vi "XP2100_Module_Manual Test_Main.vi"() -> ()   [LabVIEW 2013]
doc: "This template is for the Queued Message Handler design pattern.\n\nThe Event Handling Loop generates messages based on user interface actions.\n\nThe Message Handling Loop processes messages generated by the Event Handling Loop, or by other messages. The messages are string values, so new messages can be added easily to the Message Cases case structure in the Message Handling Loop. Each message cluster can also provide an optional value for Message Data, which is a variant that can be converted to whatever message-specific data is required."
uses:
  <instrlib>/niHSDIO/niHSDIO.llb/niHSDIO_ctl Voltage Logic Family Values (Ring).ctl
  <instrlib>/niDCPower/nidcpower.llb/niDCPower Sense.ctl
  Controls/Reg_Address_Data.ctl
  Controls/USID.ctl
  controls/UI Data.ctl
  support/Message Queue/Enqueue Message (Single).vi
  support/Message Queue/Enqueue Message (Array).vi
  <vilib>/Utility/error.llb/Error Cluster From Error Code.vi
  <vilib>/ErrorRing/Error Ring.xnode
  support/Message Queue/Message Queue.lvlib
  support/User Event - Stop/User Event - Stop.lvlib
panel:
  in  "Measure":bool=TRUE
  in  "Tab Control":T1(tab)
  in  "DUT and Bridge SMU Settings":T3={"SMU Settings"={"CH"={"voltage level range"=6.0, "current limit"=0.1, "current limit range"=0.1, "voltage level "=1.8, "CH_VIO_BRIDGE"="0", "Output Enabled"=TRUE}, "CH 2"={"voltage level range"=6.0, "current limit"=0.1, "current limit range"=0.1, "voltage level "=1.8, "CH_VSU"="1", "Output Enabled"=TRUE}, "CH 3"={"voltage level range"=6.0, "current limit"=0.1, "current limit range"=0.1, "voltage level "=1.8, "CH_RFC"="2", "Output Enabled"=TRUE}, "CH 4"={"voltage level range"=6.0, "current limit"=0.1, "current limit range"=0.1, "voltage level "=1.8, "CH_NA"="3", "Output Enabled"=FALSE}}, "sense"=1008, "aperture time"=0.01666} {"aperture time" format="%.2p"; "sense" items=["Local"=1008, "Remote"=1009]; "SMU Settings"."CH 4"."voltage level" format="%#.6p"; "SMU Settings"."CH 4"."current limit range" format="%#.6p"; "SMU Settings"."CH 4"."current limit" format="%#.6p"; "SMU Settings"."CH 4"."voltage level range" format="%#.6p"; "SMU Settings"."CH 3"."voltage level" format="%#.6p"; "SMU Settings"."CH 3"."current limit range" format="%#.6p"; "SMU Settings"."CH 3"."current limit" format="%#.6p"; "SMU Settings"."CH 3"."voltage level range" format="%#.6p"; "SMU Settings"."CH 2"."voltage level" format="%#.6p"; "SMU Settings"."CH 2"."current limit range" format="%#.6p"; "SMU Settings"."CH 2"."current limit" format="%#.6p"; "SMU Settings"."CH 2"."voltage level range" format="%#.6p"; "SMU Settings"."CH"."voltage level" format="%#.6p"; "SMU Settings"."CH"."current limit range" format="%#.6p"; "SMU Settings"."CH"."current limit" format="%#.6p"; "SMU Settings"."CH"."voltage level range" format="%#.6p"}
  in  "Instrument_Visas":T4={"DUT and Bridge Power"="4145_1", "HV_SMU"="4145_0"}
  in  "HDSIO_Settings":T6={"HSDIO VISA"="6556_0", "Waveform Directory"=path "C:/Users/user/Documents/XP2100/Waveforms", "logic family "=8, "Clock Rate"=20000000.0, "channel list (Clock,Data)"="4,6"} {"Clock Rate" format="%.2p"; "logic family" items=["5.0V Logic"=5, "3.3V Logic"=6, "2.5V Logic"=7, "1.8V Logic"=8, "1.5V Logic"=80, "1.2V Logic"=81]}
  in  "Initialize Instruments":bool
  in  "Update SMU's":bool
  in  "Throw Settings: Source Current":T7={"SMU Settings"={"CH"={"Voltage Limit"=1.0, "current limit"=0.01, "Voltage limit range"=6.0, "Current level"=0.01, "CH_RF1"="0", "Output Enabled"=TRUE}, "CH"={"Voltage Limit"=1.0, "current limit"=0.01, "Voltage limit range"=6.0, "Current level"=0.01, "CH_RF2"="1", "Output Enabled"=TRUE}, "CH"={"Voltage Limit"=1.0, "current limit"=0.01, "Voltage limit range"=6.0, "Current level"=0.01, "CH_RF3"="2", "Output Enabled"=TRUE}, "CH"={"Voltage Limit"=1.0, "current limit"=0.01, "Voltage limit range"=6.0, "Current level"=0.01, "CH_RF4"="3", "Output Enabled"=TRUE}}, "sense"=1009, "aperture time"=0.01666} {"aperture time" format="%.2p"; "sense" items=["Local"=1008, "Remote"=1009]; "SMU Settings"."CH"."Current level" format="%#.6p"; "SMU Settings"."CH"."Voltage limit range" format="%#.6p"; "SMU Settings"."CH"."current limit" format="%#.6p"; "SMU Settings"."CH"."Voltage Limit" format="%#.6p"; "SMU Settings"."CH"."Current level" format="%#.6p"; "SMU Settings"."CH"."Voltage limit range" format="%#.6p"; "SMU Settings"."CH"."current limit" format="%#.6p"; "SMU Settings"."CH"."Voltage Limit" format="%#.6p"; "SMU Settings"."CH"."Current level" format="%#.6p"; "SMU Settings"."CH"."Voltage limit range" format="%#.6p"; "SMU Settings"."CH"."current limit" format="%#.6p"; "SMU Settings"."CH"."Voltage Limit" format="%#.6p"; "SMU Settings"."CH"."Current level" format="%#.6p"; "SMU Settings"."CH"."Voltage limit range" format="%#.6p"; "SMU Settings"."CH"."current limit" format="%#.6p"; "SMU Settings"."CH"."Voltage Limit" format="%#.6p"}
  in  "Test Script w_Triggers":bool
  in  "Test Script":string="Script Lowpower\nWait until scriptTrigger0\nGenerate U13LowPower\nend Script"
  in  "RFFE Function":enum16{"Write", "Read"}(ring)
  in  "Reg_Address_Data":T8={"Address"=81, "Data"=0} {"Data" min=1; "Address" format="%.0x"}
  in  "USID":T9 max=15
  out "Read Data":cluster{"USID":u8, "Register":u8, "Data":u8} {"Register" max=31 format="%.0x"; "USID" max=15}
  in  "Run RFFE Waveform":bool
  out "Ext_Read_Reg":i32[](array[numeric])
  out "Ext_Read_Data":u8[](array[numeric])=[31, 144, 7]
  in  "Run Script":bool
  in  "Script Steps":string="\tGenerate\tBRGu8r1Cd56\n\tWait 20\t\n\tGenerate\tBRGu8r0d13\n\tWait 20\t\n\tGenerate\tBRGu8r4d7\n\tWait 20\t\n\tGenerate\tBRGu8rCd1\n\tWait 20\t\n\tGenerate\tBRGu8r3d46\n\tWait 20\t\n\tGenerate\tBRGu8r2Bd4\n\tWait 20\t\n\tGenerate\tBRGu8r4d103\n\tWait 20\t\n\tGenerate\tBRGu8r2d27\n\tWait 20\t\n\tGenerate\tBRGu8r5d9\n\tWait 20\t\n\tGenerate\tBRGu8r6d187\n\tWait 20\t\n\tGenerate\tBRGu8r7d4\n\tWait 20\t\n\tGenerate\tBRGu8r3d110\n\tWait 20\t\n\tGenerate\tBRGu8r1d184\n\tWait 20\t\n\tGenerate\tBRGu8r80d2\n\tWait 20\t\n\tGenerate\tBRGu8r4Ad242\n\tWait 20\t\n\tGenerate\tBRGu8r4Bd249\n\tWait 20\t\n\tGenerate\tBRGu8r4Dd244\n\tWait 20\t\n\tGenerate\tBRGu8rC1d253\n\twait 20\n\tGenerate \tBRGu2rAd133\n\twait 20\n\tGenerate \tBRGu8r4Dd254\n\twait 20\n\tGenerate \tBRGu8rC1d241\n\twait 20\n\tGenerate \tBRGu8rC1d247\n\twait 400"
  out "Dut and Bridge Measurements":T10 {"current measurements" format="%#_6p"}
  in  "Script Notepad: Initialize Bridge":string="\tGenerate\tBRGu8r1Cd56\n\tWait 20\t\n\tGenerate\tBRGu8r0d13\n\tWait 20\t\n\tGenerate\tBRGu8r4d7\n\tWait 20\t\n\tGenerate\tBRGu8rCd1\n\tWait 20\t\n\tGenerate\tBRGu8r3d46\n\tWait 20\t\n\tGenerate\tBRGu8r2Bd4\n\tWait 20\t\n\tGenerate\tBRGu8r4d103\n\tWait 20\t\n\tGenerate\tBRGu8r2d27\n\tWait 20\t\n\tGenerate\tBRGu8r5d9\n\tWait 20\t\n\tGenerate\tBRGu8r6d187\n\tWait 20\t\n\tGenerate\tBRGu8r7d4\n\tWait 20\t\n\tGenerate\tBRGu8r3d110\n\tWait 20\t\n\tGenerate\tBRGu8r1d184\n\tWait 20\t\n\tGenerate\tBRGu8r80d2\n\tWait 20\t\n\tGenerate\tBRGu8r4Ad242\n\tWait 20\t\n\tGenerate\tBRGu8r4Bd249\n\tWait 20\t\n\tGenerate\tBRGu8r4Dd244\n\tWait 20\t\n\tGenerate\tBRGu8rC1d253\n\twait 20\n\tGenerate \tBRGu2rAd133\n\twait 20\n\tGenerate \tBRGu8r4Dd254\n\twait 20\n\tGenerate \tBRGu8rC1d241\n\twait 20\n\tGenerate \tBRGu8rC1d247\n\twait 400"
  in  "DUT Info":T11={"Lot #"="", "Wafer #"="", "DUT Coordinates"="", "Comments"="generate HV29"}
  in  "Path":path=path "C:/Users/er080167/Desktop/Delete"
  in  "Save Button":bool
  out "USIDs_Detected":u8[](array[numeric])
  in  "Scan USID's":bool
  out "Throw Measurements":T10 {"current measurements" format="%#_6p"}
  out "Throw_Resitances":dbl[](array[numeric]) format="%#_6p"
  out "4_CH_SMU_Settings_Readback":T12(array[cluster]) {"sense 2" items=["Local"=1008, "Remote"=1009]}
  out "Write or Read":digitalwaveform(graph)={"t0"=timestamp(3585852840.1106524 s since 1904-01-01), "dt"=5e-07, "Y"={"transitions"=[], "data"=[[1, 0, 1, 0], [1, 0, 1, 0], [1, 0, 1, 0], [1, 0, 1, 0], [1, 0, 1, 0], [1, 0, 1, 0], [1, 0, 1, 0], [1, 0, 1, 0], [0, 0, 0, 0], [0, 0, 0, 0], [0, 0, 0, 0], [0, 0, 0, 0], [0, 0, 0, 0], [0, 0, 0, 0], [0, 0, 0, 0], [0, 0, 0, 0], [0, 1, 0, 1], [0, 1, 0, 1], [0, 1, 0, 1], [0, 1, 0, 1], [0, 0, 0, 0], [0, 0, 0, 0], [0, 0, 0, 0], [0, 0, 0, 0], [1, 1, 1, 1], [1, 1, 1, 1], [1, 1, 1, 1], [1, 1, 1, 1], [1, 0, 1, 0], [1, 0, 1, 0], [1, 0, 1, 0], [1, 0, 1, 0], [1, 1, 1, 1], [1, 1, 1, 1], [1, 1, 1, 1], [1, 1, 1, 1], [1, 0, 1, 0], [1, 0, 1, 0], [1, 0, 1, 0], [1, 0, 1, 0], [0, 1, 0, 1], [0, 1, 0, 1], [0, 1, 0, 1], [0, 1, 0, 1], [0, 0, 0, 0], [0, 0, 0, 0], [0, 0, 0, 0], [0, 0, 0, 0], [0, 1, 0, 1], [0, 1, 0, 1], [0, 1, 0, 1], [0, 1, 0, 1], [0, 0, 0, 0], [0, 0, 0, 0], [0, 0, 0, 0], [0, 0, 0, 0], [1, 1, 1, 1], [1, 1, 1, 1], [1, 1, 1, 1], [1, 1, 1, 1], [1, 0, 1, 0], [1, 0, 1, 0], [1, 0, 1, 0], [1, 0, 1, 0], [0, 1, 0, 1], [0, 1, 0, 1], [0, 1, 0, 1], [0, 1, 0, 1], [0, 0, 0, 0], [0, 0, 0, 0], [0, 0, 0, 0], [0, 0, 0, 0], [1, 1, 1, 1], [1, 1, 1, 1], [1, 1, 1, 1], [1, 1, 1, 1], [1, 0, 1, 0], [1, 0, 1, 0], [1, 0, 1, 0], [1, 0, 1, 0], [1, 1, 1, 1], [1, 1, 1, 1], [1, 1, 1, 1], [1, 1, 1, 1], [1, 0, 1, 0], [1, 0, 1, 0], [1, 0, 1, 0], [1, 0, 1, 0], [1, 1, 1, 1], [1, 1, 1, 1], [1, 1, 1, 1], [1, 1, 1, 1], [1, 0, 1, 0], [1, 0, 1, 0], [1, 0, 1, 0], [1, 0, 1, 0], [0, 1, 0, 1], [0, 1, 0, 1], [0, 1, 0, 1], [0, 1, 0, 1], [0, 0, 0, 0], [0, 0, 0, 0], [0, 0, 0, 0], [0, 0, 0, 0], [0, 1, 0, 1], [0, 1, 0, 1], [0, 1, 0, 1], [0, 1, 0, 1], [0, 0, 0, 0], [0, 0, 0, 0], [0, 0, 0, 0], [0, 0, 0, 0], [1, 1, 1, 1], [1, 1, 1, 1], [1, 1, 1, 1], [1, 1, 1, 1], [1, 0, 1, 0], [1, 0, 1, 0], [1, 0, 1, 0], [1, 0, 1, 0], [1, 1, 1, 1], [1, 1, 1, 1], [1, 1, 1, 1], [1, 1, 1, 1], [1, 0, 1, 0], [1, 0, 1, 0], [1, 0, 1, 0], [1, 0, 1, 0], [0, 1, 0, 1], [0, 1, 0, 1], [0, 1, 0, 1], [0, 1, 0, 1], [0, 0, 0, 0], [0, 0, 0, 0], [0, 0, 0, 0], [0, 0, 0, 0], [0, 1, 0, 1], [0, 1, 0, 1], [0, 1, 0, 1], [0, 1, 0, 1], [0, 0, 0, 0], [0, 0, 0, 0], [0, 0, 0, 0], [0, 0, 0, 0], [0, 1, 0, 1], [0, 1, 0, 1], [0, 1, 0, 1], [0, 1, 0, 1], [0, 0, 0, 0], [0, 0, 0, 0], [0, 0, 0, 0], [0, 0, 0, 0], [0, 1, 0, 1], [0, 1, 0, 1], [0, 1, 0, 1], [0, 1, 0, 1], [0, 0, 0, 0], [0, 0, 0, 0], [0, 0, 0, 0], [0, 0, 0, 0], [0, 1, 0, 1], [0, 1, 0, 1], [0, 1, 0, 1], [0, 1, 0, 1], [0, 0, 0, 0], [0, 0, 0, 0], [0, 0, 0, 0], [0, 0, 0, 0], [0, 1, 0, 1], [0, 1, 0, 1], [0, 1, 0, 1], [0, 1, 0, 1], [0, 0, 0, 0], [0, 0, 0, 0], [0, 0, 0, 0], [0, 0, 0, 0], [0, 1, 0, 1], [0, 1, 0, 1], [0, 1, 0, 1], [0, 1, 0, 1], [0, 0, 0, 0], [0, 0, 0, 0], [0, 0, 0, 0], [0, 0, 0, 0], [0, 1, 0, 1], [0, 1, 0, 1], [0, 1, 0, 1], [0, 1, 0, 1], [0, 0, 0, 0], [0, 0, 0, 0], [0, 0, 0, 0], [0, 0, 0, 0], [0, 1, 0, 1], [0, 1, 0, 1], [0, 1, 0, 1], [0, 1, 0, 1], [0, 0, 0, 0], [0, 0, 0, 0], [0, 0, 0, 0], [0, 0, 0, 0], [1, 0, 1, 0], [1, 0, 1, 0], [1, 0, 1, 0], [1, 0, 1, 0], [1, 0, 1, 0], [1, 0, 1, 0], [1, 0, 1, 0], [1, 0, 1, 0], [0, 0, 0, 0], [0, 0, 0, 0], [0, 0, 0, 0], [0, 0, 0, 0], [0, 0, 0, 0], [0, 0, 0, 0], [0, 0, 0, 0], [0, 0, 0, 0], [0, 1, 0, 1], [0, 1, 0, 1], [0, 1, 0, 1], [0, 1, 0, 1], [0, 0, 0, 0], [0, 0, 0, 0], [0, 0, 0, 0], [0, 0, 0, 0], [1, 1, 1, 1], [1, 1, 1, 1], [1, 1, 1, 1], [1, 1, 1, 1], [1, 0, 1, 0], [1, 0, 1, 0], [1, 0, 1, 0], [1, 0, 1, 0], [1, 1, 1, 1], [1, 1, 1, 1], [1, 1, 1, 1], [1, 1, 1, 1], [1, 0, 1, 0], [1, 0, 1, 0], [1, 0, 1, 0], [1, 0, 1, 0], [0, 1, 0, 1], [0, 1, 0, 1], [0, 1, 0, 1], [0, 1, 0, 1], [0, 0, 0, 0], [0, 0, 0, 0], [0, 0, 0, 0], [0, 0, 0, 0], [0, 1, 0, 1], [0, 1, 0, 1], [0, 1, 0, 1], [0, 1, 0, 1], [0, 0, 0, 0], [0, 0, 0, 0], [0, 0, 0, 0], [0, 0, 0, 0], [1, 1, 1, 1], [1, 1, 1, 1], [1, 1, 1, 1], [1, 1, 1, 1], [1, 0, 1, 0], [1, 0, 1, 0], [1, 0, 1, 0], [1, 0, 1, 0], [1, 1, 1, 1], [1, 1, 1, 1], [1, 1, 1, 1], [1, 1, 1, 1], [1, 0, 1, 0], [1, 0, 1, 0], [1, 0, 1, 0], [1, 0, 1, 0], [1, 1, 1, 1], [1, 1, 1, 1], [1, 1, 1, 1], [1, 1, 1, 1], [1, 0, 1, 0], [1, 0, 1, 0], [1, 0, 1, 0], [1, 0, 1, 0], [1, 1, 1, 1], [1, 1, 1, 1], [1, 1, 1, 1], [1, 1, 1, 1], [1, 0, 1, 0], [1, 0, 1, 0], [1, 0, 1, 0], [1, 0, 1, 0], [1, 1, 1, 1], [1, 1, 1, 1], [1, 1, 1, 1], [1, 1, 1, 1], [1, 0, 1, 0], [1, 0, 1, 0], [1, 0, 1, 0], [1, 0, 1, 0], [0, 1, 0, 1], [0, 1, 0, 1], [0, 1, 0, 1], [0, 1, 0, 1], [0, 0, 0, 0], [0, 0, 0, 0], [0, 0, 0, 0], [0, 0, 0, 0], [0, 1, 0, 1], [0, 1, 0, 1], [0, 1, 0, 1], [0, 1, 0, 1], [0, 0, 0, 0], [0, 0, 0, 0], [0, 0, 0, 0], [0, 0, 0, 0], [0, 1, 0, 1], [0, 1, 0, 1], [0, 1, 0, 1], [0, 1, 0, 1], [0, 0, 0, 0], [0, 0, 0, 0], [0, 0, 0, 0], [0, 0, 0, 0], [0, 1, 0, 1], [0, 1, 0, 1], [0, 1, 0, 1], [0, 1, 0, 1], [0, 0, 0, 0], [0, 0, 0, 0], [0, 0, 0, 0], [0, 0, 0, 0], [1, 1, 5, 1], [1, 1, 5, 1], [1, 1, 5, 1], [1, 1, 5, 1], [1, 0, 4, 0], [1, 0, 5, 0], [1, 0, 5, 0], [1, 0, 5, 0], [0, 1, 5, 1], [0, 1, 5, 1], [0, 1, 5, 1], [0, 1, 5, 1], [0, 0, 3, 0], [0, 0, 5, 0], [0, 0, 5, 0], [0, 0, 5, 0], [0, 1, 5, 1], [0, 1, 5, 1], [0, 1, 5, 1], [0, 1, 5, 1], [0, 0, 3, 0], [0, 0, 5, 0], [0, 0, 5, 0], [0, 0, 5, 0], [0, 1, 5, 1], [0, 1, 5, 1], [0, 1, 5, 1], [0, 1, 5, 1], [0, 0, 3, 0], [0, 0, 5, 0], [0, 0, 5, 0], [0, 0, 5, 0], [0, 1, 5, 1], [0, 1, 5, 1], [0, 1, 5, 1], [0, 1, 5, 1], [0, 0, 3, 0], [0, 0, 5, 0], [0, 0, 5, 0], [0, 0, 5, 0], [0, 1, 5, 1], [0, 1, 5, 1], [0, 1, 5, 1], [0, 1, 5, 1], [0, 0, 3, 0], [0, 0, 5, 0], [0, 0, 5, 0], [0, 0, 5, 0], [0, 1, 5, 1], [0, 1, 5, 1], [0, 1, 5, 1], [0, 1, 5, 1], [0, 0, 3, 0], [0, 0, 5, 0], [0, 0, 5, 0], [0, 0, 5, 0], [0, 1, 5, 1], [0, 1, 5, 1], [0, 1, 5, 1], [0, 1, 5, 1], [0, 0, 3, 0], [0, 0, 5, 0], [0, 0, 5, 0], [0, 0, 5, 0], [0, 1, 5, 1], [0, 1, 5, 1], [0, 1, 5, 1], [0, 1, 5, 1], [0, 0, 3, 0], [0, 0, 5, 0], [0, 0, 5, 0], [0, 0, 5, 0], [0, 1, 0, 1], [0, 1, 0, 1], [0, 1, 0, 1], [0, 1, 0, 1], [0, 0, 0, 0], [0, 0, 0, 0], [0, 0, 0, 0], [0, 0, 0, 0]]}}
  out "Throw_4_CH_SMU_Settings_Readback":T12(array[cluster]) {"sense 2" items=["Local"=1008, "Remote"=1009]}
  out "Display <Replace Me>":string="\"Exit\" button pressed"
  in  "Exit":bool
  # "CH_VIO_BRIDGE"
  # "CH_VSU"
  # "CH_RFC"
  # "CH_NA"
  # "CH_VIO_BRIDGE"
  # "CH_VSU"
  # "CH_VP"
  # "CH_DUT_VIO"
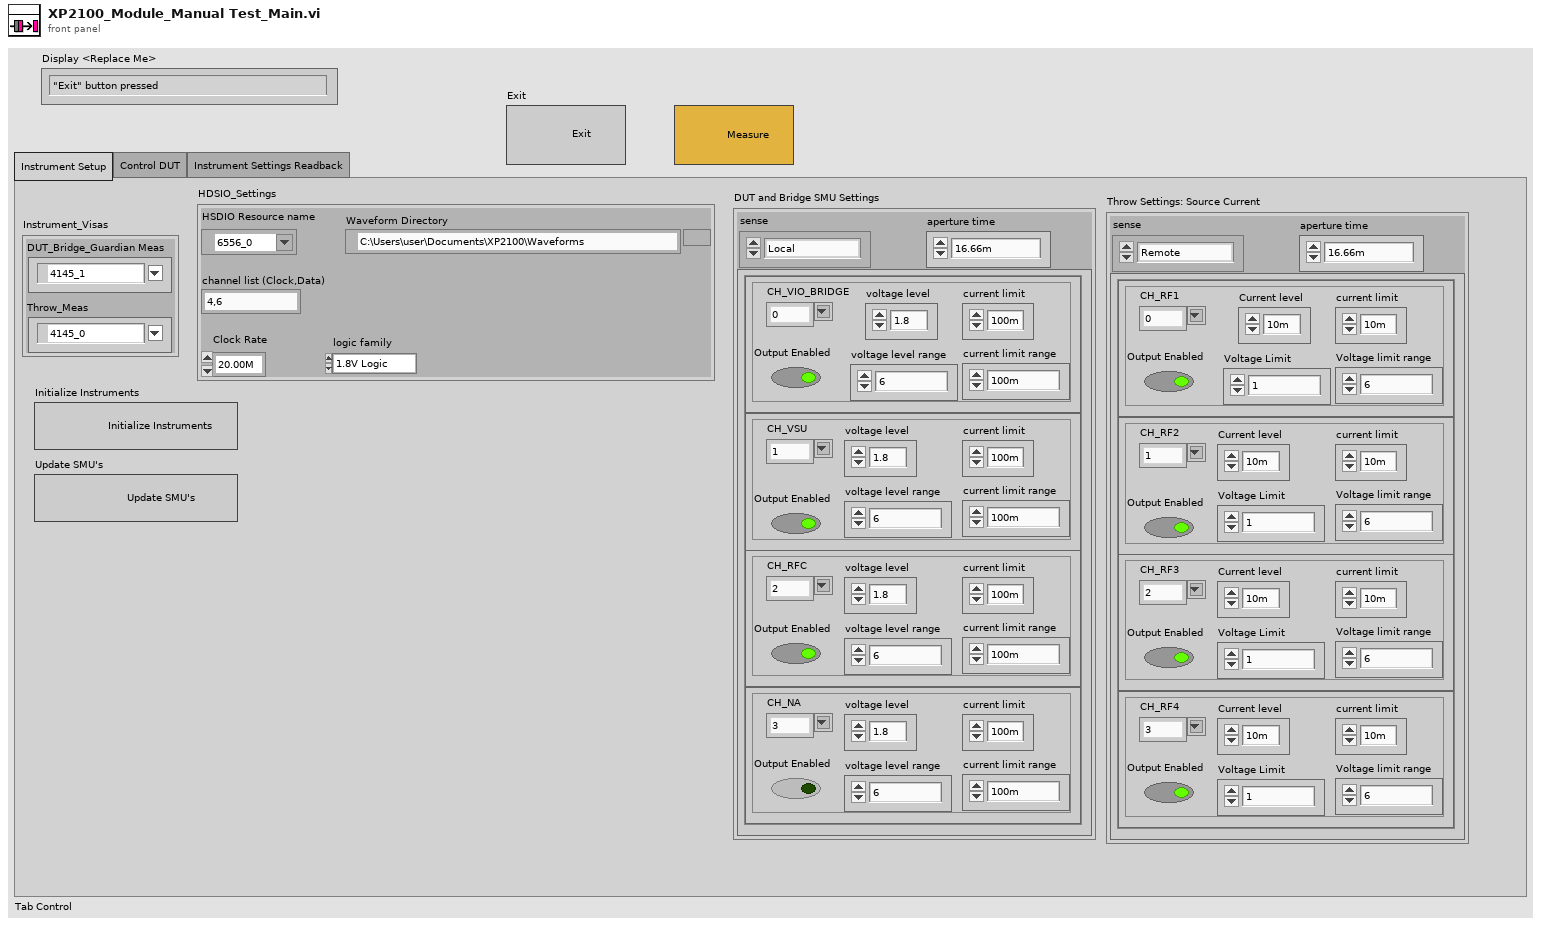
[diagram p1: front panel]
types:
  T1 = enum32{"Instrument Setup", "Control DUT", "Instrument Settings Readback"}
  T2 = typedef "niDCPower Sense.ctl" = i32
  T3 = cluster{"SMU Settings":cluster{"CH":cluster{"voltage level range":dbl, "current limit":dbl, "current limit range":dbl, "voltage level ":dbl, "CH_VIO_BRIDGE":string, "Output Enabled":bool}, "CH 2":cluster{"voltage level range":dbl, "current limit":dbl, "current limit range":dbl, "voltage level ":dbl, "CH_VSU":string, "Output Enabled":bool}, "CH 3":cluster{"voltage level range":dbl, "current limit":dbl, "current limit range":dbl, "voltage level ":dbl, "CH_RFC":string, "Output Enabled":bool}, "CH 4":cluster{"voltage level range":dbl, "current limit":dbl, "current limit range":dbl, "voltage level ":dbl, "CH_NA":string, "Output Enabled":bool}}, "sense":T2, "aperture time":dbl}
  T4 = cluster{"DUT and Bridge Power":refnum<k15>, "HV_SMU":refnum<k15>}
  T5 = typedef "niHSDIO_ctl Voltage Logic Family Values (Ring).ctl" = i32
  T6 = cluster{"HSDIO VISA":refnum<k15>, "Waveform Directory":path, "logic family ":T5, "Clock Rate":dbl, "channel list (Clock,Data)":string}
  T7 = cluster{"SMU Settings":cluster{"CH":cluster{"Voltage Limit":dbl, "current limit":dbl, "Voltage limit range":dbl, "Current level":dbl, "CH_RF1":string, "Output Enabled":bool}, "CH":cluster{"Voltage Limit":dbl, "current limit":dbl, "Voltage limit range":dbl, "Current level":dbl, "CH_RF2":string, "Output Enabled":bool}, "CH":cluster{"Voltage Limit":dbl, "current limit":dbl, "Voltage limit range":dbl, "Current level":dbl, "CH_RF3":string, "Output Enabled":bool}, "CH":cluster{"Voltage Limit":dbl, "current limit":dbl, "Voltage limit range":dbl, "Current level":dbl, "CH_RF4":string, "Output Enabled":bool}}, "sense":T2, "aperture time":dbl}
  T8 = typedef "Reg_Address_Data.ctl" = cluster{"Address":u8, "Data":u8}
  T9 = typedef "USID.ctl" = u8
  T10 = cluster{"voltage measurements":dbl[], "current measurements":dbl[]}
  T11 = cluster{"Lot #":string, "Wafer #":string, "DUT Coordinates":string, "Comments":string}
  T12 = cluster{"Source Range":dbl, "Source Limit":dbl, "Source  limit range":dbl, "Source level":dbl, "CH":string, "Output Enabled":bool, "Source Mode":enum16{"Voltage", "Current"}, "aperture time":dbl, "sense 2":T2}[]
  T13 = cluster{"HV SMU Settings":cluster{"Source Range":dbl, "Source Limit":dbl, "Source  limit range":dbl, "Source level":dbl, "CH":string, "Output Enabled":bool, "Source Mode":enum16{"Voltage", "Current"}, "aperture time":dbl, "sense 2":T2}, "PI<0>":cluster{"Source Range":dbl, "Source Limit":dbl, "Source  limit range":dbl, "Source level":dbl, "CH":string, "Output Enabled":bool, "Source Mode":enum16{"Voltage", "Current"}, "aperture time":dbl, "sense 2":T2}}
  T14 = cluster{"SMU Settings":cluster{"CH":cluster{"voltage level range":dbl, "current limit":dbl, "current limit range":dbl, "voltage level ":dbl, "CH_VIO_BRIDGE":string, "Output Enabled":bool}, "CH 2":cluster{"voltage level range":dbl, "current limit":dbl, "current limit range":dbl, "voltage level ":dbl, "CH_VSU":string, "Output Enabled":bool}, "CH 3":cluster{"voltage level range":dbl, "current limit":dbl, "current limit range":dbl, "voltage level ":dbl, "CH_VP":string, "Output Enabled":bool}, "CH 4":cluster{"voltage level range":dbl, "current limit":dbl, "current limit range":dbl, "voltage level ":dbl, "CH_DUT_VIO":string, "Output Enabled":bool}}, "sense":T2, "aperture time":dbl}
  T15 = cluster{"HSDIO_ACQ":refnum<k15>, "HSDIO_GEN":refnum<k15>}
  T16 = typedef "UI Data.ctl" = cluster{"Boolean <Replace Me>":bool, "String <Replace Me>":string, "Numeric <Replace Me>":dbl, "Do Something Ref":refnum<vi>, "Do Something Else Ref":refnum<vi>, "Data Display Ref":refnum<vi>, "Exit Button Ref":refnum<vi>}
  T17 = typedef "Message Queue.lvlib/All Message Queues.ctl" = cluster{"UI":refnum<queue>}
  T18 = cluster{"First Reg Address":u8, "Num of Reg to Read":u8}
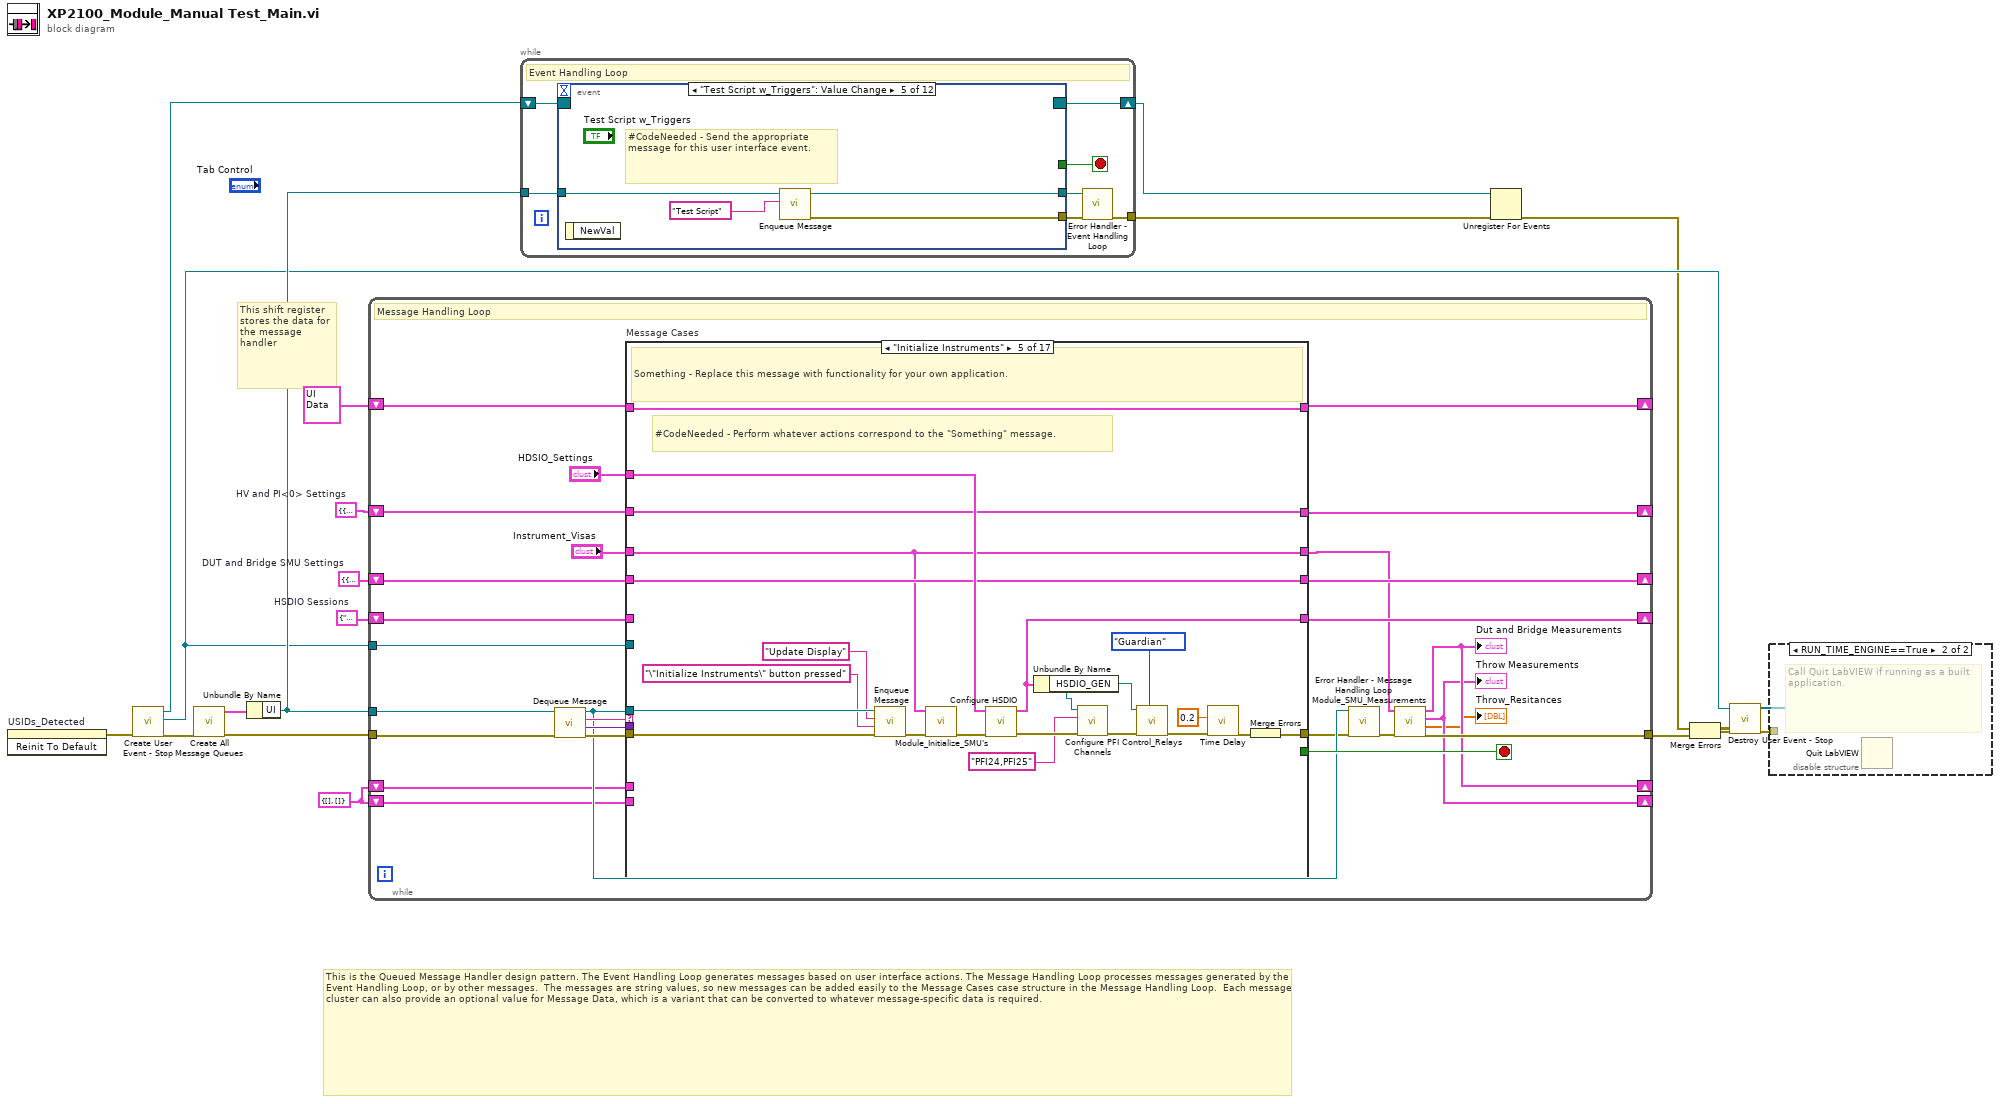
[diagram p0: block diagram]
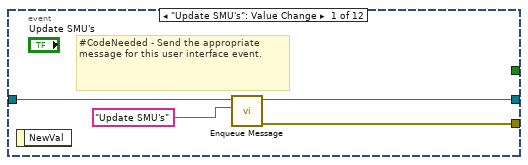
[diagram p3: hidden frame]
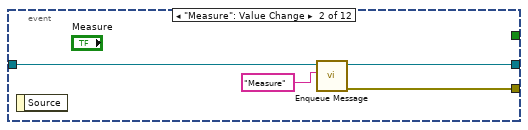
[diagram p4: hidden frame]
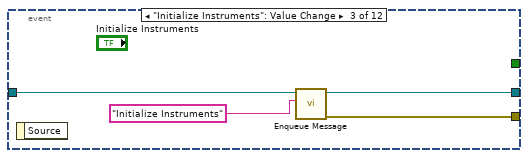
[diagram p5: hidden frame]
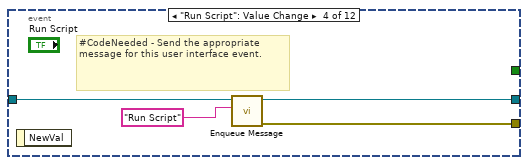
[diagram p6: hidden frame]
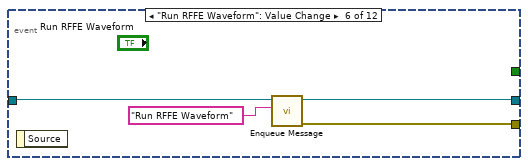
[diagram p7: hidden frame]
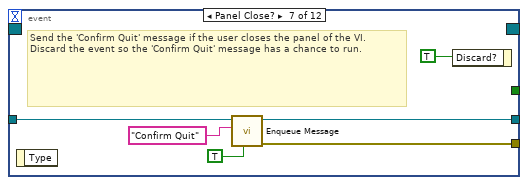
[diagram p8: hidden frame]
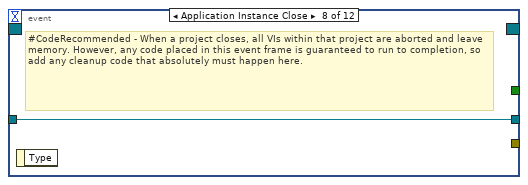
[diagram p9: hidden frame]
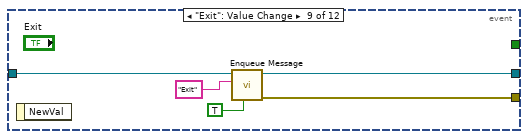
[diagram p10: hidden frame]
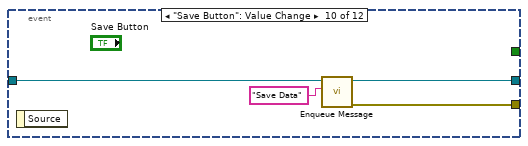
[diagram p11: hidden frame]
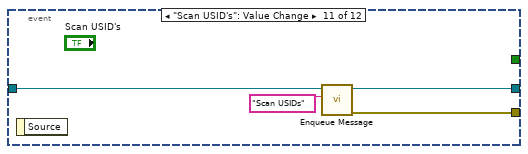
[diagram p12: hidden frame]
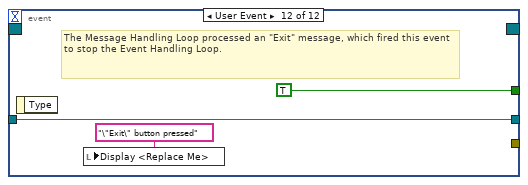
[diagram p13: hidden frame]
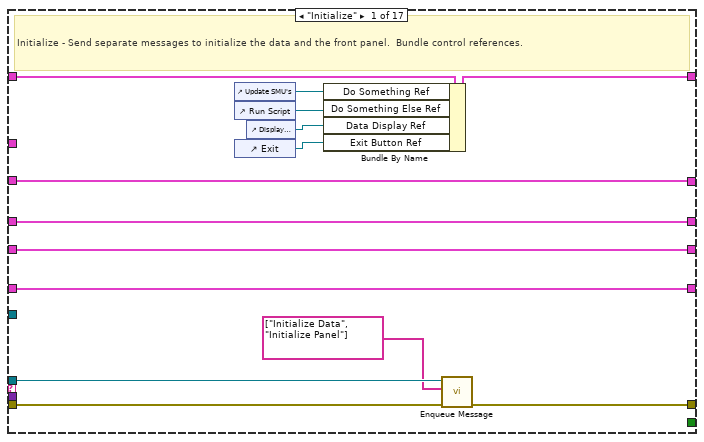
[diagram p14: hidden frame]
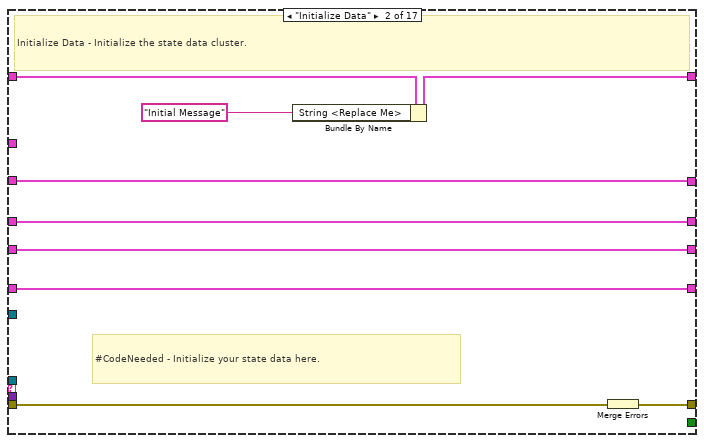
[diagram p15: hidden frame]
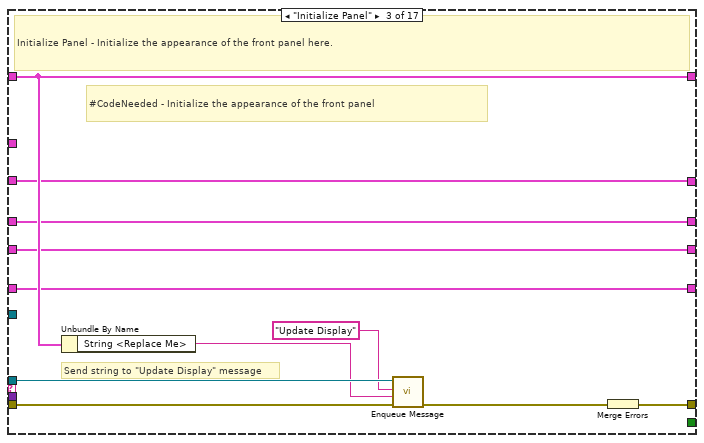
[diagram p16: hidden frame]
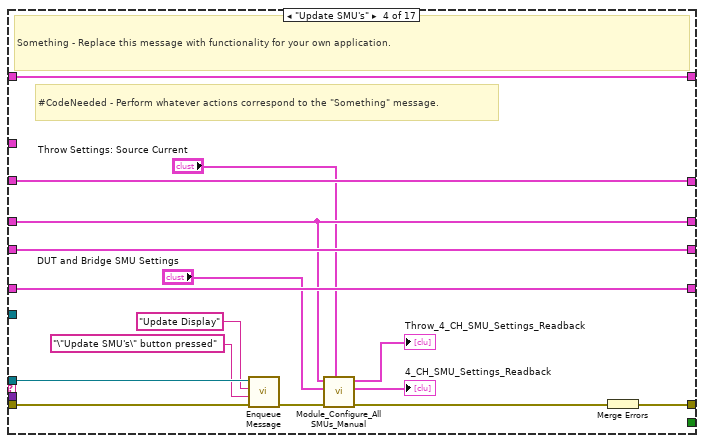
[diagram p17: hidden frame]
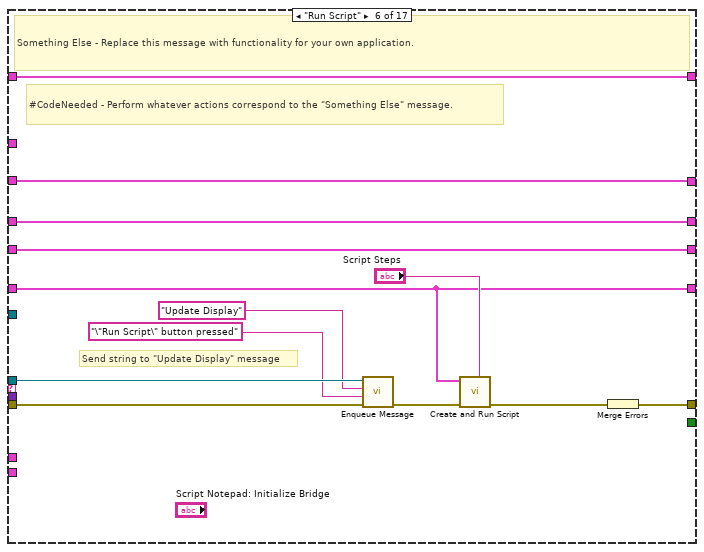
[diagram p18: hidden frame]
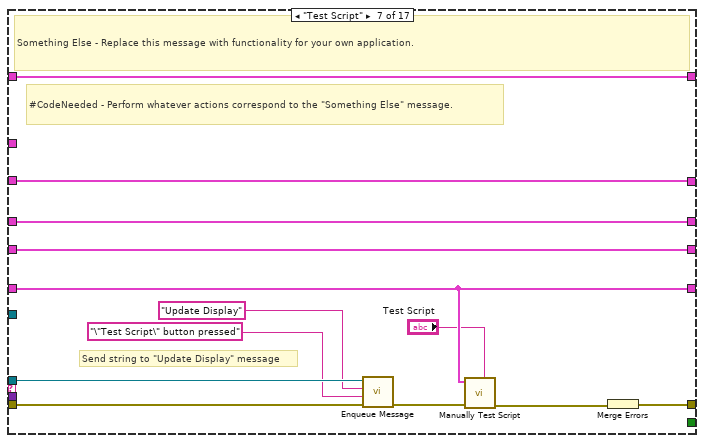
[diagram p19: hidden frame]
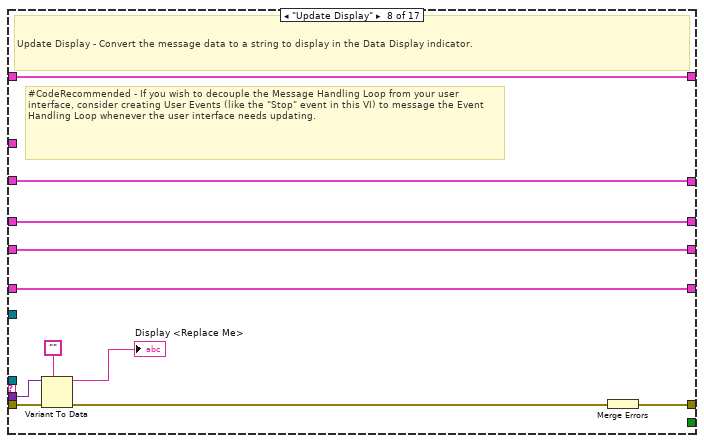
[diagram p20: hidden frame]
diagram:
  w1 = T13 {"HV SMU Settings"={"Source Range"=0.0001, "Source Limit"=60.0, "Source  limit range"=60.0, "Source level"=0.0, "CH"="0", "Output Enabled"=FALSE, "Source Mode"=enum."Current", "aperture time"=0.001, "sense 2"=1009}, "PI<0>"={"Source Range"=6.0, "Source Limit"=0.01, "Source  limit range"=0.01, "Source level"=1.2, "CH"="0", "Output Enabled"=FALSE, "Source Mode"=enum."Voltage", "aperture time"=0.01666, "sense 2"=1009}}  # HV and PI<0> Settings
  w2 = T14 {"SMU Settings"={"CH"={"voltage level range"=0.0, "current limit"=0.0, "current limit range"=0.0, "voltage level "=0.0, "CH_VIO_BRIDGE"="", "Output Enabled"=FALSE}, "CH 2"={"voltage level range"=0.0, "current limit"=0.0, "current limit range"=0.0, "voltage level "=0.0, "CH_VSU"="", "Output Enabled"=FALSE}, "CH 3"={"voltage level range"=0.0, "current limit"=0.0, "current limit range"=0.0, "voltage level "=0.0, "CH_VP"="", "Output Enabled"=FALSE}, "CH 4"={"voltage level range"=0.0, "current limit"=0.0, "current limit range"=0.0, "voltage level "=0.0, "CH_DUT_VIO"="", "Output Enabled"=FALSE}}, "sense"=0, "aperture time"=0.0}  # DUT and Bridge SMU Settings
  w5 = T10 {"voltage measurements"=[], "current measurements"=[]} ("PI<0> Measurements")
  w6 = T15 {"HSDIO_ACQ"="", "HSDIO_GEN"=""}  # HSDIO Sessions
  # "This is the Queued Message Handler design pattern. The Event Handling Loop generates messages based on user interface actions. The Message Handling Loop processes messages generated by the Event Handling Loop, or by other messages.  The messages are string values, so new messages can be added easily to the Message Cases case structure in the Message Handling Loop.  Each message cluster can also provide an optional value for Message Data, which is a variant that can be converted to whatever message-specific data is required."
  # "This shift register stores the data for the message handler"
  n1 = invoke on="USIDs_Detected" class="Arr (strict)" method="Reinit To Default"() -> (error out=w3:errorcluster)  [unwired: 3 in, 2 out]
  n2 = call "Create User Event - Stop.vi"("error in (no error)"=w3) -> ("error out"=w14:errorcluster, "User Event - Stop"=w12:refnum<user-event>, "Stop Event Registration Refnum"=w15:refnum<event-registration>)  [unwired: 8 in]
  n3 = call "Create All Message Queues.vi"("error in (no error)"=w14) -> ("error out"=w4:errorcluster, "Message Queues out"=w18:T17)  [unwired: 9 in]
  n4 = Unbundle By Name(w18) -> ("UI"=w16:refnum<queue>)
  n5 = while {
    tunnel: w16 -> [w37]
    shift-right: [w44] -> _
    shift-left: T16 {"Boolean <Replace Me>"=FALSE, "String <Replace Me>"="", "Numeric <Replace Me>"=0.0, "Do Something Ref"=refnum, "Do Something Else Ref"=refnum, "Data Display Ref"=refnum, "Exit Button Ref"=refnum} ("Data Cluster") -> [w45]
    tunnel: w12 -> [w42]
    tunnel: w4 -> [w41]
    tunnel: [w23] -> w17
    shift-right: [w32] -> _
    shift-left: w6 -> [w31]
    shift-right: [w20] -> _
    shift-left: w5 -> [w29]
    shift-right: [w21] -> _
    shift-left: w5 -> [w30]
    shift-right: [w28] -> _
    shift-left: w2 -> [w27]
    shift-right: [w26] -> _
    shift-left: w1 -> [w25]
    stop <- w43 stop-if-true
    # "Message Handling Loop"
    n6 = call "Dequeue Message.vi"("error in (no error)"=w41, "Message Queue"=w37) -> ("error out"=w40:errorcluster, "Message Data"=w38:variant, "Message"=w39:string, "dup Message Queue"=w36:refnum<queue>)  [unwired: 6 in]
    n7 = case "Message Cases" shown="\"Initialize Instruments\"" w39 {
      selector: w39 -> [_ _ _ _ _ _ _ _ _ _ _ _ _ _ _ _ w260]
      tunnel: w36 -> [w57 _ w76 w93 w114 w126 w139 _ w160 w175 _ _ _ _ w236 w255 _]
      tunnel: w40 -> [w58 w68 w77 w90 w111 w127 w140 w151 w168 w179 w186 w193 w207 w218 w237 w251 _]
      tunnel: [w59 w64 w78 w94 w115 w128 w141 w152 w161 w177 w184 w191 w209 w221 w240 w248 w261] -> w35
      tunnel: w45 -> [w56 w67 w79 w95 w116 w129 w142 w153 w167 w178 w185 w192 w210 w222 w241 w254 w262]
      tunnel: [w55 w66 w79 w95 w116 w129 w142 w153 w167 w178 w185 w192 w210 w222 w241 w254 w262] -> w44
      tunnel: [_ _ _ _ _ _ _ _ _ _ _ _ _ _ _ TRUE _] -> w43
      tunnel: w38 -> [_ _ _ _ _ _ _ w150 w166 _ _ _ _ _ _ _ _]
      tunnel: w42 -> [_ _ _ _ _ _ _ _ _ _ _ _ _ _ _ w250 _]
      tunnel: w25 -> [w47 w61 w70 w87 w107 w118 w131 w144 w154 w170 w181 w188 w201 w212 w224 w246 w257]
      tunnel: "Instrument_Visas" -> [w49 w62 w72 w81 w105 w123 w136 w146 w157 w171 w183 w190 w208 w220 w225 w242 w259]
      tunnel: [w49 w62 w72 w81 w105 w123 w136 w146 w157 w171 w183 w190 w208 w220 w225 w242 w259] -> w22
      tunnel: "HDSIO_Settings" -> [_ _ _ _ w110 _ _ _ _ _ _ _ _ _ _ _ _]
      tunnel: [w48 w63 w71 w89 w101 w119 w133 w145 w156 w172 w182 w189 w206 w219 w226 w247 w258] -> w32
      tunnel: w31 -> [w48 w63 w71 w89 _ w119 w133 w145 w156 w172 w182 w189 w206 w219 w226 w247 w258]
      tunnel: w30 -> [_ _ _ _ _ _ _ _ _ _ _ _ _ w214 _ _ _]
      tunnel: w29 -> [_ _ _ _ _ _ _ _ _ _ _ _ _ w213 _ _ _]
      tunnel: [w46 w60 w69 w88 w106 w117 w130 w143 w155 w169 w180 w187 w200 w211 w223 w245 w256] -> w28
      tunnel: w27 -> [w46 w60 w69 w88 w106 w117 w130 w143 w155 w169 w180 w187 w200 w211 w223 w245 w256]
      tunnel: [w47 w61 w70 w87 w107 w118 w131 w144 w154 w170 w181 w188 w201 w212 w224 w246 w257] -> w26
      frame "Initialize" {
        # "Initialize - Send separate messages to initialize the data and the front panel.  Bundle control references."
        n8 = control-ref of="Update SMU's"() -> (w54:refnum<vi>)
        n9 = control-ref of="Run Script"() -> (w53:refnum<vi>)
        n10 = control-ref of="Exit"() -> (w51:refnum<vi>)
        n11 = control-ref of="Display <Replace Me>"() -> (w52:refnum<vi>)
        n12 = Bundle By Name(cluster=w56, "Do Something Ref"=w54, "Do Something Else Ref"=w53, "Data Display Ref"=w52, "Exit Button Ref"=w51) -> (w55:T16)
        n13 = call-poly "Enqueue Message.vi"("error in (no error)"=w58, "Message Array"=string[] ["Initialize Data", "Initialize Panel"], "Message Queue"=w57) -> ("error out"=w59:errorcluster)  [unwired: 7 in, 1 out]
      }
      frame "Initialize Data" {
        # "#CodeNeeded - Initialize your state data here."
        # "Initialize Data - Initialize the state data cluster."
        n14 = Bundle By Name(cluster=w67, "String <Replace Me>"="Initial Message" ("Initial Message")) -> (w66:T16)
        n15 = Merge Errors(w68) -> (w64:errorcluster)
      }
      frame "Initialize Panel" {
        # "Send string to \"Update Display\" message"
        # "#CodeNeeded - Initialize the appearance of the front panel"
        # "Initialize Panel - Initialize the appearance of the front panel here."
        n16 = Unbundle By Name(w79) -> ("String <Replace Me>"=w73:string)
        n17 = call-poly "Enqueue Message.vi"("error in (no error)"=w77, "Message Data"=w73, "Message"="Update Display", "Message Queue"=w76) -> ("error out"=w75:errorcluster)  [unwired: 6 in, 1 out]
        n18 = Merge Errors(w75) -> (w78:errorcluster)
      }
      frame "Update SMU's" {
        # "#CodeNeeded - Perform whatever actions correspond to the \"Something\" message."
        # "Something - Replace this message with functionality for your own application."
        n19 = call-poly "Enqueue Message.vi"("error in (no error)"=w90, "Message Data"="\"Update SMU's\" button pressed" ("\"Do Something\" button pressed"), "Message"="Update Display", "Message Queue"=w93) -> ("error out"=w85:errorcluster)  [unwired: 6 in, 1 out]
        n20 = call "Module_Configure_All SMUs_Manual.vi"("Throw Settings"="Throw Settings: Source Current", "Error In"=w85, "DUT and Bridge SMU Settings"="DUT and Bridge SMU Settings", "Instrument_Visas"=w81) -> ("Error Out"=w84:errorcluster, "DUR_4_CH_SMU"=→"4_CH_SMU_Settings_Readback":T12, "Throw_4_CH_SMU"=→"Throw_4_CH_SMU_Settings_Readback":T12)  [unwired: 5 in]
        n21 = Merge Errors(w84) -> (w94:errorcluster)
      }
      frame "Initialize Instruments" {
        # "#CodeNeeded - Perform whatever actions correspond to the \"Something\" message."
        # "Something - Replace this message with functionality for your own application."
        n22 = call-poly "Enqueue Message.vi"("error in (no error)"=w111, "Message Data"="\"Initialize Instruments\" button pressed" ("\"Do Something\" button pressed"), "Message"="Update Display", "Message Queue"=w114) -> ("error out"=w104:errorcluster)  [unwired: 6 in, 1 out]
        n23 = call "Module_Initialize_SMU's.vi"("Error In"=w104, "Instrument_Visas"=w105) -> ("Error Out"=w103:errorcluster)  [unwired: 9 in]
        n24 = call "Configure HSDIO.vi"("error in (no error)"=w103, "HDSIO_Settings"=w110) -> ("error out"=w102:errorcluster, "HSDIO Sessions"=w101:T15)  [unwired: 8 in]
        n25 = Unbundle By Name(w101) -> ("HSDIO_GEN"=w96:refnum<k15>)
        n26 = call "Configure PFI Channels.vi"("Error In"=w102, "channel list (all:\"\")"="PFI24,PFI25" ("channel list (all:\"\")"), "instrument handle"=w96) -> ("Error Out"=w99:errorcluster)  [unwired: 8 in]
        n27 = call "Control_Relays.vi"("Test_Configuration"=enum16{"Throws", "Guardian"}."Guardian", "Error In"=w99, "instrument handle"=w96) -> ("Error Out"=w98:errorcluster)  [unwired: 8 in]
        n28 = call "Time Delay"("error in (no error)"=w98, "Delay Time (s)"=0.2) -> ("error out"=w109:errorcluster)  [unwired: 9 in]
        n29 = Merge Errors(w109) -> (w115:errorcluster)
      }
      frame "Run Script" {
        # "Send string to \"Update Display\" message"
        # "#CodeNeeded - Perform whatever actions correspond to the \"Something Else\" message."
        # "Something Else - Replace this message with functionality for your own application."
        n30 = call-poly "Enqueue Message.vi"("error in (no error)"=w127, "Message Data"="\"Run Script\" button pressed" ("\"Do Something Else\" button pressed"), "Message"="Update Display", "Message Queue"=w126) -> ("error out"=w121:errorcluster)  [unwired: 6 in, 1 out]
        n31 = call "Create and Run Script.vi"("Script Steps"="Script Steps", "Error In"=w121, "HSDIO Sessions"=w119) -> ("Error Out"=w120:errorcluster)  [unwired: 8 in]
        n32 = Merge Errors(w120) -> (w128:errorcluster)
      }
      frame "Test Script" {
        # "Send string to \"Update Display\" message"
        # "#CodeNeeded - Perform whatever actions correspond to the \"Something Else\" message."
        # "Something Else - Replace this message with functionality for your own application."
        n33 = call-poly "Enqueue Message.vi"("error in (no error)"=w140, "Message Data"="\"Test Script\" button pressed" ("\"Do Something Else\" button pressed"), "Message"="Update Display", "Message Queue"=w139) -> ("error out"=w135:errorcluster)  [unwired: 6 in, 1 out]
        n34 = call "Manually Test Script.vi"("Copy Script Into Window"="Test Script", "Error In"=w135, "HSDIO Sessions"=w133) -> ("Error Out"=w134:errorcluster)  [unwired: 8 in]
        n35 = Merge Errors(w134) -> (w141:errorcluster)
      }
      frame "Update Display" {
        # "#CodeRecommended - If you wish to decouple the Message Handling Loop from your user interface, consider creating User Events (like the \"Stop\" event in this VI) to message the Event Handling Loop whenever the user interface needs updating."
        # "Update Display - Convert the message data to a string to display in the Data Display indicator."
        n36 = Variant To Data(error in=w151, type="", Variant=w150) -> (data=→"Display <Replace Me>":string, error out=w148:errorcluster)
        n37 = Merge Errors(w148) -> (w152:errorcluster)
      }
      frame "Error" {
        # "#CodeRecommended - If you ever change the name of this \"Error\" message, you'll need to update the name in the Check Loop Error.vi as well."
        # "#CodeRecommended - This code will always pop up an error dialog and call the 'Exit' message if an error occurs. Add more fine-grained error handling here."
        # "Error - Check the error message data and respond accordingly. This message is sent by the \"Error Handler\" VIs at the end of each loop in this application."
        n38 = Variant To Data(error in=w168, type=errorcluster {"status"=FALSE, "code"=0, "source"=""} ("error constant"), Variant=w166) -> (data=w164:errorcluster, error out=w163:errorcluster)
        n39 = call <vilib>:"Simple Error Handler.vi"("error in (no error)"=w164) -> ()  [unwired: 4 in, 5 out]
        n40 = call-poly "Enqueue Message.vi"("Priority Message? (F)"=TRUE, "Message"="Exit", "Message Queue"=w160) -> ("error out"=w162:errorcluster)  [unwired: 7 in, 1 out]
        n41 = Merge Errors(w162, w163) -> (w161:errorcluster)
      }
      frame "Confirm Quit" {
        # "#CodeNeeded - If you want to provide an \"Are you sure\" dialog (or some other notification) before the application exits, place that code here. This message is typically sent from a Panel Close? event."
        # "Confirm Quit - Message that can confirm whether or not the user wants to exit the application."
        n42 = call-poly "Enqueue Message.vi"("Priority Message? (F)"=TRUE, "error in (no error)"=w179, "Message"="Exit", "Message Queue"=w175) -> ("error out"=w176:errorcluster)  [unwired: 6 in, 1 out]
        n43 = Merge Errors(w176) -> (w177:errorcluster)
      }
      frame "---Copy This Frame---" {
        # "Duplicate this frame when creating new messages.  Change this comment in the duplicated frame to describe this message."
        n44 = Merge Errors(w186) -> (w184:errorcluster)
      }
      frame "Measure" {
        # "Duplicate this frame when creating new messages.  Change this comment in the duplicated frame to describe this message."
        n45 = Merge Errors(w193) -> (w191:errorcluster)
      }
      frame "Scan USIDs" {
        w204 = T9[] [1, 2, 4, 7, 8, 9, 13, 15]  # Potential_USID_Array
        # "USID 8 is Bridge Default"
        # "Duplicate this frame when creating new messages.  Change this comment in the duplicated frame to describe this message."
        n46 = call "Bridge_SCAN_USIDs.vi"("HSDIO Sessions"=w206, "Potential_USID_Array"=w204, "Error In"=w207, "Reg_Address_to_Read"=T18 {"First Reg Address"=31, "Num of Reg to Read"=1}) -> ("USIDs_Detected"=w198:u8[], "Error Out"=w203:errorcluster)  [unwired: 11 in, 3 out]
        "USIDs_Detected" <- w198
        n47 = Search 1D Array(1D array=w198, element=u8 8) -> (index of element=w197:i32)  [unwired: 1 in]
        n48 = Delete From Array(array=w198, index=w197) -> (array with subset deleted=w196:u8[])  [unwired: 1 in, 1 out]
        n49 = Index Array(array=w196, index=0) -> (element=w194:u8)
        n50 = property on="USID" class="DigNum (strict)"(error in=w203, "Value"=w194) -> (error out=w202:errorcluster)  [unwired: 1 in, 1 out]
        n51 = Merge Errors(w202) -> (w209:errorcluster)
      }
      frame "Save Data" {
        # "Duplicate this frame when creating new messages.  Change this comment in the duplicated frame to describe this message."
        n52 = call "Save Data.vi"("HV Measurements"=w213, "Error In"=w218, "Dut and Bridge Measurements"=w214, "DUT Info"="DUT Info", "Path"="Path") -> ("error out"=w217:errorcluster)  [unwired: 6 in]
        n53 = Merge Errors(w217) -> (w221:errorcluster)
      }
      frame "Run RFFE Waveform" {
        # "Duplicate this frame when creating new messages.  Change this comment in the duplicated frame to describe this message."
        n54 = call-poly "Enqueue Message.vi"("error in (no error)"=w237, "Message Data"="\"Run RFFE Waveform\" button pressed" ("\"Do Something Else\" button pressed"), "Message"="Update Display", "Message Queue"=w236) -> ("error out"=w234:errorcluster)  [unwired: 6 in, 1 out]
        n55 = call "RFFE Main Control.vi"("RFFE Function"="RFFE Function", "Error In"=w234, "Reg_Address_Data"="Reg_Address_Data", "USID"="USID", "HSDIO Sessions"=w226) -> ("Error Out"=w235:errorcluster, "Converted Data"=→"Read Data":cluster{"USID":u8, "Register":u8, "Data":u8}, "Data_Readback"=→"Ext_Read_Data":u8[], "Registers_Readback"=→"Ext_Read_Reg":i32[], "HSDIO"=→"Write or Read":digitalwaveform)  [unwired: 2 in]
        n56 = Merge Errors(w235) -> (w240:errorcluster)
      }
      frame "Exit" {
        # "Stop the VI"
        # "Release the message queue reference"
        # "#CodeNeeded - Add any required cleanup code here"
        # "Exit - Exit the application."
        n57 = call "Fire User Event - Stop.vi"("User Event - Stop"=w250) -> ("error out"=w249:errorcluster)  [unwired: 10 in]
        n58 = Release Queue(queue=w255, error in (no error)=w251) -> (error out=w252:errorcluster)  [unwired: 1 in, 2 out]
        n59 = Merge Errors(w249, w252) -> (w244:errorcluster)
        n60 = call "Module_Close_SMU's.vi"("Error In"=w244, "Instrument_Visas"=w242) -> ("Error Out"=w243:errorcluster)  [unwired: 9 in]
        n61 = call "CLOSE_HSDIO.vi"("Error In"=w243, "HSDIO Sessions"=w247) -> ("Error Out"=w248:errorcluster)  [unwired: 9 in]
      }
      frame Default {
        # "'Default' case only runs if there is a message that isn't defined in any of the other cases.  Output a programming error."
        n62 = xnode "Error Ring"("parameter 0"=w260) -> ("error out"=w261:errorcluster)
      }
    }
    n63 = call "Error Handler - Message Handling Loop.vi"("error in (no error)"=w35, "Message Queue"=w36) -> ("dup error in"=w24:errorcluster)  [unwired: 8 in, 1 out]
    n64 = call "Module_SMU_Measurements.vi"("Error In"=w24, "Instrument_Visas"=w22) -> ("Error Out"=w23:errorcluster, "Throw_Resitances"=→"Throw_Resitances":dbl[], "Throw Measurements"=w20:T10, "Dut and Bridge Measurements"=w21:T10)  [unwired: 6 in]
    "Dut and Bridge Measurements" <- w21
    "Throw Measurements" <- w20
  }
  n65 = while {
    tunnel: w16 -> [w276]
    shift-right: [w274] -> w10
    shift-left: w15 -> [w275]
    tunnel: [w270] -> w7
    stop <- w272 stop-if-true
    # "Event Handling Loop"
    n66 = event shown="[4] \"Test Script w_Triggers\": Value Change" {
      selector: w275 -> [_ _ _ _ _ _ _ _ _ _ _ _]
      dyn-events: [_ _ _ _ _ _ _ _ _ _ _ _] -> w274
      timeout: _ -> [_ _ _ _ _ _ _ _ _ _ _ _]
      tunnel: [_ _ _ _ _ _ _ _ _ _ _ TRUE ("Discard?")] -> w272
      tunnel: w276 -> [w280 w284 w287 w292 w296 w299 w305 w307 w312 w316 w320 w323]
      tunnel: [w277 w281 w288 w289 w293 w297 w304 _ w311 w314 w318 _] -> w273
      tunnel: [w279 w283 w286 w291 w295 w298 w303 w307 w310 w315 w319 w323] -> w271
      event "Update SMU's": Value Change {
        # "#CodeNeeded - Send the appropriate message for this user interface event."
        n67 = event-data() -> ()  [unwired: 1 in, 1 out]
        n68 = call-poly "Enqueue Message.vi"("Message"="Update SMU's", "Message Queue"=w280) -> ("error out"=w277:errorcluster, "dup Message Queue"=w279:refnum<queue>)  [unwired: 8 in]
      }
      event "Measure": Value Change {
        n69 = event-data() -> ()  [unwired: 1 in, 1 out]
        n70 = call-poly "Enqueue Message.vi"("Message"="Measure", "Message Queue"=w284) -> ("error out"=w281:errorcluster, "dup Message Queue"=w283:refnum<queue>)  [unwired: 8 in]
      }
      event "Initialize Instruments": Value Change {
        n71 = event-data() -> ()  [unwired: 1 in, 1 out]
        n72 = call-poly "Enqueue Message.vi"("Message"="Initialize Instruments", "Message Queue"=w287) -> ("error out"=w288:errorcluster, "dup Message Queue"=w286:refnum<queue>)  [unwired: 8 in]
      }
      event "Run Script": Value Change {
        # "#CodeNeeded - Send the appropriate message for this user interface event."
        n73 = event-data() -> ()  [unwired: 1 in, 1 out]
        n74 = call-poly "Enqueue Message.vi"("Message"="Run Script", "Message Queue"=w292) -> ("error out"=w289:errorcluster, "dup Message Queue"=w291:refnum<queue>)  [unwired: 8 in]
      }
      event "Test Script w_Triggers": Value Change {
        # "#CodeNeeded - Send the appropriate message for this user interface event."
        n75 = event-data() -> ()  [unwired: 1 in, 1 out]
        n76 = call-poly "Enqueue Message.vi"("Message"="Test Script", "Message Queue"=w296) -> ("error out"=w293:errorcluster, "dup Message Queue"=w295:refnum<queue>)  [unwired: 8 in]
      }
      event "Run RFFE Waveform": Value Change {
        n77 = event-data() -> ()  [unwired: 1 in, 1 out]
        n78 = call-poly "Enqueue Message.vi"("Message"="Run RFFE Waveform", "Message Queue"=w299) -> ("error out"=w297:errorcluster, "dup Message Queue"=w298:refnum<queue>)  [unwired: 8 in]
      }
      event Panel Close? {
        # "Send the 'Confirm Quit' message if the user closes the panel of the VI. Discard the event so the 'Confirm Quit' message has a chance to run."
        n79 = event-data() -> ()  [unwired: 1 in, 1 out]
        n80 = call-poly "Enqueue Message.vi"("Priority Message? (F)"=TRUE, "Message"="Confirm Quit", "Message Queue"=w305) -> ("error out"=w304:errorcluster, "dup Message Queue"=w303:refnum<queue>)  [unwired: 7 in]
        n81 = event-data("Discard?"=TRUE) -> ()  [unwired: 1 in, 1 out]
      }
      event Application Instance Close {
        # "#CodeRecommended - When a project closes, all VIs within that project are aborted and leave memory. However, any code placed in this event frame is guaranteed to run to completion, so add any cleanup code that absolutely must happen here."
        n82 = event-data() -> ()  [unwired: 1 in, 1 out]
      }
      event "Exit": Value Change {
        n83 = event-data() -> ()  [unwired: 1 in, 1 out]
        n84 = call-poly "Enqueue Message.vi"("Priority Message? (F)"=TRUE, "Message"="Exit", "Message Queue"=w312) -> ("error out"=w311:errorcluster, "dup Message Queue"=w310:refnum<queue>)  [unwired: 7 in]
      }
      event "Save Button": Value Change {
        n85 = event-data() -> ()  [unwired: 1 in, 1 out]
        n86 = call-poly "Enqueue Message.vi"("Message"="Save Data", "Message Queue"=w316) -> ("error out"=w314:errorcluster, "dup Message Queue"=w315:refnum<queue>)  [unwired: 8 in]
      }
      event "Scan USID's": Value Change {
        n87 = event-data() -> ()  [unwired: 1 in, 1 out]
        n88 = call-poly "Enqueue Message.vi"("Message"="Scan USIDs", "Message Queue"=w320) -> ("error out"=w318:errorcluster, "dup Message Queue"=w319:refnum<queue>)  [unwired: 8 in]
      }
      event User Event {
        # "The Message Handling Loop processed an \"Exit\" message, which fired this event to stop the Event Handling Loop."
        n89 = event-data() -> ()  [unwired: 1 in, 1 out]
        n90 = local write "Display <Replace Me>"("\"Exit\" button pressed" ("VI Stopped")) -> ()
      }
    }
    n91 = call "Error Handler - Event Handling Loop.vi"("error in (no error)"=w273, "Message Queue"=w271) -> ("dup error in"=w270:errorcluster)  [unwired: 8 in, 1 out]
  }
  n92 = Unregister For Events(event registration refnum=w10, error in=w7) -> (error out=w11:errorcluster)
  n93 = Merge Errors(w11, w17) -> (w13:errorcluster)
  n94 = call "Destroy User Event - Stop.vi"("error in (no error)"=w13, "User Event - Stop"=w12) -> ("error out"=w8:errorcluster)  [unwired: 9 in]
  n95 = disable-structure shown="RUN_TIME_ENGINE==True" {
    disable-tunnel: w8 -> [_ _]
    frame condition #0 (active) {
    }
    frame condition #1 {
      # "Call Quit LabVIEW if running as a built application."
      n96 = Quit LabVIEW() -> ()  [unwired: 1 in]
    }
  }
